vi "system.vi"(8 "Error In":errorcluster) -> (0 "Error Out":errorcluster, 2 "Value":refnum<class "QLocale.lvclass">)   [LabVIEW 2014, in "QLocale.lvclass"]
doc: "LabVIEW-specific documentation is not yet available. See <b>https://doc.qt.io/qt-5/qlocale.html#system</b>"
uses:
  QLocale.lvclass
  LQSerialData/LQSerialData.lvclass/LQSerialData.ctl
  LQ Core.lvlib
  LQSerialData/LQSerialData.lvclass
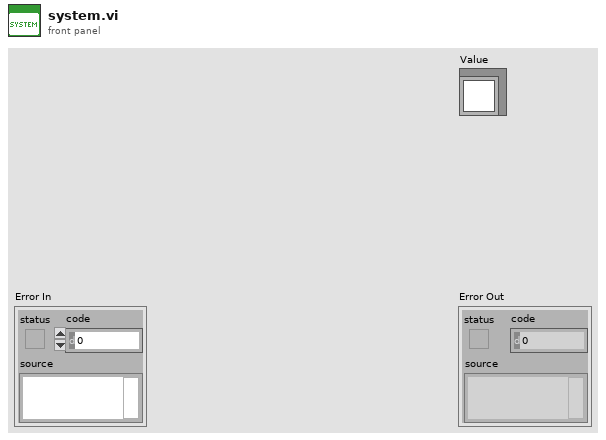
[diagram p1: front panel]
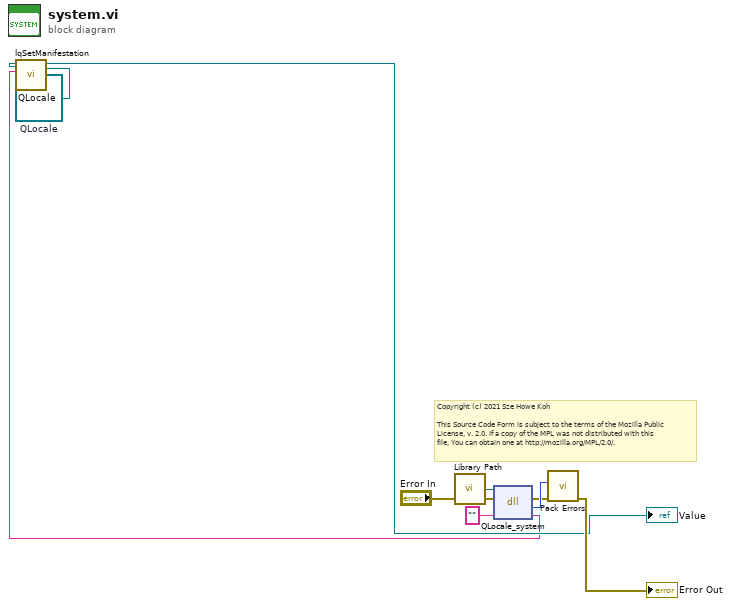
[diagram p0: block diagram]
diagram:
  w1 = refnum<class "QLocale.lvclass"> refnum  # QLocale
  # "Copyright (c) 2021 Sze Howe Koh\n\nThis Source Code Form is subject to the terms of the Mozilla Public\nLicense, v. 2.0. If a copy of the MPL was not distributed with this\nfile, You can obtain one at http://mozilla.org/MPL/2.0/."
  n1 = call "Library Path.vi"() -> ("Library Path"=w7:path)
  n2 = dll-call lib="?" fn="QLocale_system"(path in=w7, error in="Error In", "_retVal"="" ("retVal")) -> (error out=w5:errorcluster, w6:i32, "_retVal"=w2:string)  [unwired: 1 in, 1 out]
  n3 = call "lqSetManifestation.vi"("Manifestation"=w2, "LQSerialData in"=w1) -> ("LQSerialData out"=→"Value":refnum<class "QLocale.lvclass">)  [unwired: 8 in, 1 out]
  n4 = call "Pack Errors.vi"("Error In"=w5, "Error Code"=w6) -> ("Error Out"=→"Error Out":errorcluster)  [unwired: 9 in]
